vi "r-theta(deg) to XY.vi"(9 "deg [0,360]":dbl, 11 "circle radius":dbl=5.0 format="%#_13g") -> (0 "ArrayPoint[0]":cluster{"X[0]":dbl[], "Y[0]":dbl[]}, 1 "XY Point":cluster{"X":dbl, "Y":dbl}, 2 "Y":dbl, 3 "X":dbl)   [LabVIEW 2017]
doc: "Developed by Kevin Thompson\nkevin@thompsonengineering.net\n\nCopyright 2018-2020\nThompson Engineering, LLC"
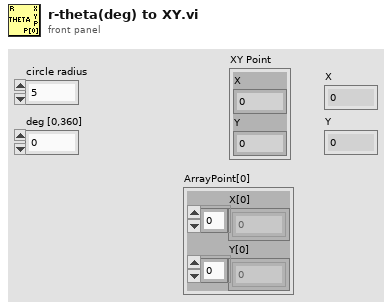
[diagram p1: front panel]
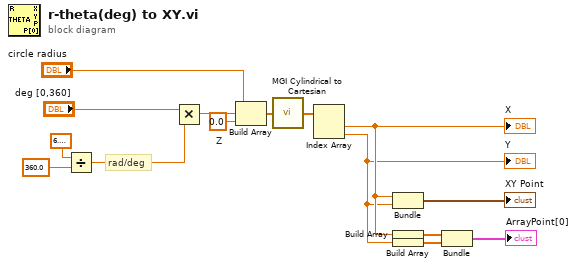
[diagram p0: block diagram]
diagram:
  w11 = 0.0  # Z
  # "rad/deg"
  n1 = Divide(x=6.283185307179586, y=360.0) -> (x/y=w8:dbl)
  n2 = Multiply(x="deg [0,360]", y=w8) -> (x*y=w15:dbl)
  n3 = Build Array("circle radius", w15, w11) -> (w13:dbl[])
  n4 = call <userlib>:"MGI Cylindrical to Cartesian.vi"("R,Th,Z"=w13) -> ("X,Y,Z"=w14:dbl[])
  n5 = Index Array(array=w14) -> (element #1=w3:dbl, element #2=w2:dbl)  [unwired: 2 in]
  "X" <- w3
  "Y" <- w2
  n6 = Bundle("Numeric"=w3, "Numeric"=w2) -> (→"XY Point":cluster{"Numeric":dbl, "Numeric":dbl})  [unwired: 1 in]
  n7 = Build Array(w3) -> (w4:dbl[])
  n8 = Build Array(w2) -> (w5:dbl[])
  n9 = Bundle(w4, w5) -> (→"ArrayPoint[0]":cluster{dbl[], dbl[]})  [unwired: 1 in]
